vi "Actor Event.vi"(8 "Queue Mailbox":refnum<data-value>, 9 "Self Event Alias":string, 10 "Queue of Self Event":refnum<queue>, 11 "Event":refnum<class "Event.lvclass">) -> ()   [LabVIEW 2021, in "jettl.lvlib" / "Base Event.lvlib" / "Base Event.lvclass"]
uses:
  Base Event.lvclass
  Self Event/Self Event.lvlib
  Event/Event.lvclass
  jettl.lvlib
  Last Ack Created Event Msg Strategy/Last Ack Created Event Msg Strategy.lvlib
  C:/git/jettl/jettl/jettl/jettl/jettl.lvclass
  C:/git/jettl/jettl/Merge Error Msg Strategy/Merge Error/Merge Error.lvclass
  C:/git/jettl/jettl/jettl/Event/Event.lvclass
  C:/git/jettl/jettl/jettl/Last Ack Creator Queue Msg Strategy/Last Ack Creator Queue/Last Ack Creator Queue.lvclass
  C:/git/jettl/jettl/Override Error Msg Strategy/Override Error/Override Error.lvclass
  C:/git/jettl/jettl/Set Panel State Msg Strategy/Set Panel State/Set Panel State.lvclass
  C:/git/jettl/jettl/Setup Msg Strategy/Setup/Setup.lvclass
  C:/git/jettl/jettl/Teardown Msg Strategy/Teardown/Teardown.lvclass
  C:/git/jettl/jettl/jettl/Base Event/Base Event/Base Event.lvclass
  Msg Strategy/Msg Strategy.lvclass
  Queue Mailbox/Queue Mailbox/Queue Mailbox.lvclass
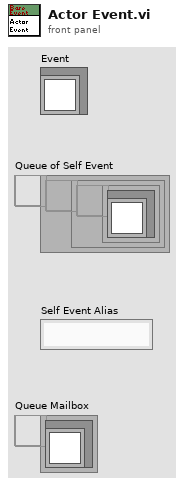
[diagram p1: front panel]
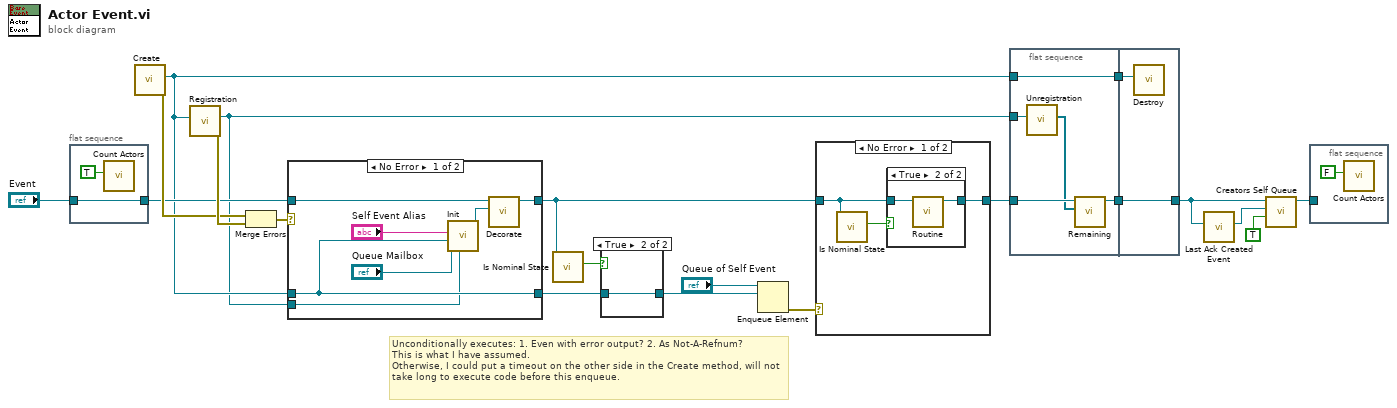
[diagram p0: block diagram]
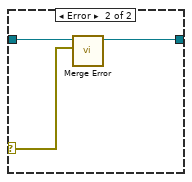
[diagram p3: hidden frame]
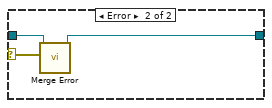
[diagram p5: hidden frame]
diagram:
  # "Unconditionally executes: 1. Even with error output? 2. As Not-A-Refnum?\nThis is what I have assumed.\nOtherwise, I could put a timeout on the other side in the Create method, will not take long to execute code before this enqueue."
  n1 = flat-sequence {
    tunnel: [w21] -> w16
    tunnel: "Event" -> [w21]
    frame #0 {
      n2 = call "Count Actors.vi"("Increment?"=TRUE) -> ()  [unwired: 11 in]
    }
  }
  n3 = call "Create.vi"() -> ("error out"=w19:errorcluster, "Self Event"=w11:refnum<data-value>)  [unwired: 10 in]
  n4 = call "Registration.vi"("Self Event"=w11) -> ("error out"=w20:errorcluster, "Registration"=w8:refnum<event-registration>)  [unwired: 9 in]
  n5 = Merge Errors(w19, w20) -> (w18:errorcluster)
  n6 = case shown="No Error" w18 {
    selector: w18 -> [_ w31]
    tunnel: [w27 w32] -> w3
    tunnel: w16 -> [w29 w30]
    tunnel: w11 -> [w24 _]
    tunnel: [w24 _] -> w5
    tunnel: w8 -> [w23 _]
    frame No Error {
      n7 = call "Init.vi"("Registration"=w23, "Queue Mailbox"="Queue Mailbox", "Self Event"=w24, "Self Event Alias"="Self Event Alias") -> ("Base Event out"=w28:refnum<class "Base Event.lvclass">)  [unwired: 7 in]
      n8 = call-dynamic "Decorate.vi"("Event"=w28, "Event in"=w29) -> ("Event out"=w27:refnum<class "Event.lvclass">)  [unwired: 9 in]
    }
    frame Error {
      n9 = call-dynamic "Merge Error.vi"("Error"=w31, "Merge Error in"=w30) -> ("Merge Error out"=w32:refnum<class "Event.lvclass">)  [unwired: 9 in]
    }
  }
  n10 = call-dynamic "Is Nominal State.vi"("jettl in"=w3) -> ("Is Nominal State?"=w6:bool)  [unwired: 10 in]
  n11 = case shown="True" w6 {
    tunnel: [_ w33] -> w4
    tunnel: w5 -> [_ w33]
    frame False {
    }
    frame True {
    }
  }
  n12 = Enqueue Element(queue="Queue of Self Event", element=w4) -> (error out=w1:errorcluster)  [unwired: 2 in, 2 out]
  n13 = case shown="No Error" w1 {
    selector: w1 -> [_ w40]
    tunnel: [w36 w41] -> w2
    tunnel: w3 -> [w34 w42]
    frame No Error {
      n14 = call-dynamic "Is Nominal State.vi"("jettl in"=w34) -> ("Is Nominal State?"=w35:bool)  [unwired: 10 in]
      n15 = case shown="True" w35 {
        tunnel: w34 -> [w37 w39]
        tunnel: [w37 w38] -> w36
        frame False {
        }
        frame True {
          n16 = call-dynamic "Routine.vi"("jettl in"=w39) -> ("jettl out"=w38:refnum<class "Event.lvclass">)  [unwired: 10 in]
        }
      }
    }
    frame Error {
      n17 = call-dynamic "Merge Error.vi"("Error"=w40, "Merge Error in"=w42) -> ("Merge Error out"=w41:refnum<class "Event.lvclass">)  [unwired: 9 in]
    }
  }
  n18 = flat-sequence {
    tunnel: w8 -> [w46]
    tunnel: w2 -> [w45]
    tunnel: w11 -> [w47]
    tunnel: [w47] -> w10
    tunnel: [w44] -> w9
    tunnel: [w48] -> w12
    tunnel: w10 -> [w49]
    tunnel: w9 -> [w48]
    frame #0 {
      n19 = call "Unregistration.vi"("Registration"=w46) -> ("Remaining"=w43:refnum<class "Msg Strategy.lvclass">[])  [unwired: 10 in]
      n20 = call-dynamic "Remaining.vi"("Remaining"=w43, "jettl in"=w45) -> ("jettl out"=w44:refnum<class "Event.lvclass">)  [unwired: 9 in]
    }
    frame #1 {
      n21 = call "Destroy.vi"("Self Event"=w49) -> ()  [unwired: 10 in, 1 out]
    }
  }
  n22 = call "Last Ack Created Event.vi"("Event"=w12) -> ("Msg Strategy"=w14:refnum<class "Msg Strategy.lvclass">)  [unwired: 10 in]
  n23 = call-dynamic "Creators Self Queue.vi"("Priority?"=TRUE, "Msg Strategy"=w14, "Event in"=w12) -> ("Event out"=w7:refnum<class "Event.lvclass">)  [unwired: 8 in]
  n24 = flat-sequence {
    tunnel: w7 -> [_]
    frame #0 {
      n25 = call "Count Actors.vi"("Increment?"=FALSE) -> ()  [unwired: 11 in]
    }
  }
